vi "channel_setenv.vi"() -> ()   [LabVIEW 2017]
doc: "Illustrates how to set an environment variable in the remote channel's process space and read it back using 'printenv'."
uses:
  libssh2/libssh2_session_handshake_tcp.vi
  libssh2/libssh2_init_default.vi
  libssh2/libssh2_session_init_ex.vi
  <vilib>/Utility/tcp.llb/TCP Get Raw Net Object.vi
  libssh2/libssh2_session_handshake_socket.vi
  libssh2/libssh2_userauth_password_ex.vi
  libssh2/libssh2_channel_open_ex.vi
  libssh2/libssh2_channel_process_startup.vi
  libssh2/libssh2_channel_read_ex.vi
  libssh2/libssh2.lvlib
panel:
  in  "value":string="Hello, World!"
  in  "varname":string="MY_VAR"
  out "Output":string
  in  "password":string
  in  "username":string
  out "error out":errorcluster
  in  "hostname":string="localhost"
  # "Note:\nBefore you can set an environment variable on your SSH server,\nmake sure to add your variable to the AcceptEnv configuration\nof your SSH server.\n\nFor example:\nAcceptEnv MY_*"
  # "printenv:\nhttps://www.man7.org/linux/man-pages/man1/printenv.1.html"
  # "AcceptEnv:\nhttps://www.man7.org/linux/man-pages/man5/sshd_config.5.html"
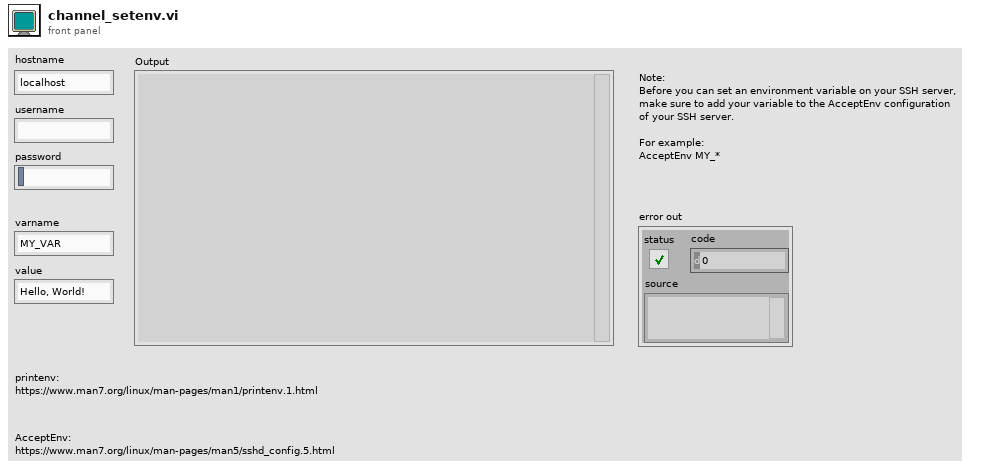
[diagram p1: front panel]
types:
  T1 = typedef "libssh2.lvlib/Session Refnum.ctl" = refnum<k1>
  T2 = typedef "libssh2.lvlib/Channel Refnum.ctl" = refnum<k1>
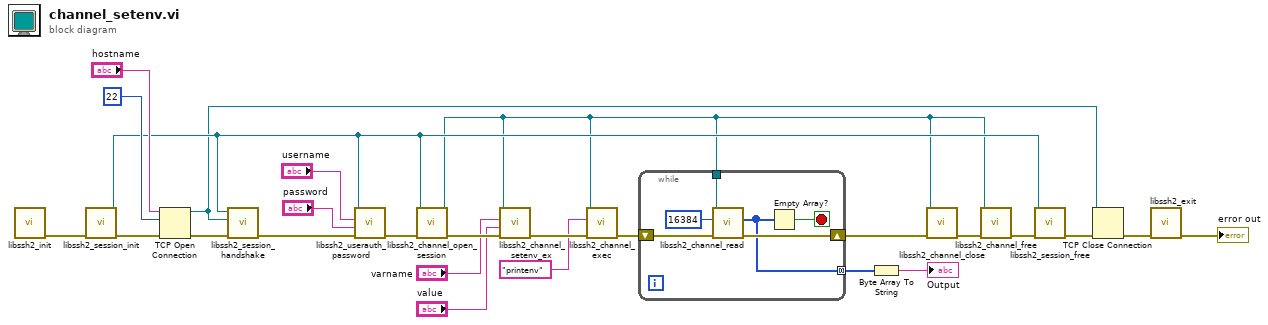
[diagram p0: block diagram]
diagram:
  n1 = call-poly "libssh2_init.vi"() -> ("error out"=w26:errorcluster)  [unwired: 11 in]
  n2 = call "libssh2_session_init.vi"("error in (no error)"=w26) -> ("error out"=w25:errorcluster, "session"=w11:T1)  [unwired: 9 in]
  n3 = TCP Open Connection(address="hostname", remote port or service name=u16 22, error in (no error)=w25) -> (connection ID=w8:refnum<k5>, error out=w9:errorcluster)  [unwired: 2 in]
  n4 = call-poly "libssh2_session_handshake.vi"("error in (no error)"=w9, "tcp connection"=w8, "session"=w11) -> ("error out"=w7:errorcluster)  [unwired: 8 in]
  n5 = call "libssh2_userauth_password.vi"("error in (no error)"=w7, "password"="password", "username"="username", "session"=w11) -> ("error out"=w20:errorcluster)  [unwired: 7 in]
  n6 = call "libssh2_channel_open_session.vi"("error in (no error)"=w20, "session"=w11) -> ("error out"=w17:errorcluster, "channel"=w5:T2)  [unwired: 8 in]
  n7 = call "libssh2_channel_setenv_ex.vi"("error in (no error)"=w17, "value"="value", "varname"="varname", "channel"=w5) -> ("error out"=w6:errorcluster)  [unwired: 7 in]
  n8 = call "libssh2_channel_exec.vi"("error in (no error)"=w6, "command"="printenv", "channel"=w5) -> ("error out"=w16:errorcluster)  [unwired: 8 in]
  n9 = while {
    tunnel: w5 -> [w29]
    tunnel: [w27] -> w13 mode=concatenating
    shift-right: [w31] -> w15
    shift-left: w16 -> [w32]
    stop <- w28 stop-if-true
    n10 = call "libssh2_channel_read.vi"("error in (no error)"=w32, "buffer length"=16384 ("buflen"), "channel"=w29) -> ("error out"=w31:errorcluster, "buffer"=w27:u8[])  [unwired: 7 in]
    n11 = Empty Array?(array=w27) -> (empty?=w28:bool)
  }
  n12 = Byte Array To String(unsigned byte array=w13) -> (string=→"Output":string)
  n13 = call "libssh2_channel_close.vi"("error in (no error)"=w15, "channel"=w5) -> ("error out"=w1:errorcluster)  [unwired: 9 in]
  n14 = call "libssh2_channel_free.vi"("error in (no error)"=w1, "channel"=w5) -> ("error out"=w14:errorcluster)  [unwired: 9 in]
  n15 = call "libssh2_session_free.vi"("error in (no error)"=w14, "session"=w11) -> ("error out"=w24:errorcluster)  [unwired: 9 in]
  n16 = TCP Close Connection(connection ID=w8, error in (no error)=w24) -> (error out=w10:errorcluster)  [unwired: 1 in, 1 out]
  n17 = call "libssh2_exit.vi"("error in (no error)"=w10) -> ("error out"=→"error out":errorcluster)  [unwired: 10 in]
